vi "Autonomous Independent.vi"() -> ()   [LabVIEW 2016]
doc: "This VI is called when autonomous begins, and will automatically be terminated when autonomous ends. You can carry out timed or sensor driven robot movement independently without needing to return to the caller."
uses:
  <vilib>/Rock Robotics/Network Tables/NT Read Number.vi
  <vilib>/Rock Robotics/WPI/Solenoid/WPI_SolenoidValue.ctl
  Users/admin/Documents/Auto_Action_Typedef.ctl
panel:
  in  "Value":T1=enum."Forward"
  out "Auto Mode":dbl=3.0
  in  "Auton_Modes":T3(array[cluster])=[{"Actions"=[{"Effort"=0.55, "Duration"=3.5, "Action"=enum."Nothing"}, {"Effort"=0.0, "Duration"=0.0, "Action"=enum."Nothing"}]}, {"Actions"=[{"Effort"=0.0, "Duration"=1.0, "Action"=enum."Nothing"}, {"Effort"=0.75, "Duration"=5.0, "Action"=enum."Nothing"}, {"Effort"=0.0, "Duration"=1.0, "Action"=enum."Nothing"}]}, {"Actions"=[{"Effort"=1.0, "Duration"=3.0, "Action"=enum."Nothing"}, {"Effort"=0.0, "Duration"=1.0, "Action"=enum."Nothing"}, {"Effort"=0.75, "Duration"=3.5, "Action"=enum."Nothing"}, {"Effort"=0.0, "Duration"=1.0, "Action"=enum."Nothing"}]}, {"Actions"=[{"Effort"=0.0, "Duration"=0.5, "Action"=enum."Nothing"}, {"Effort"=0.8, "Duration"=5.28, "Action"=enum."Nothing"}, {"Effort"=0.0, "Duration"=1.0, "Action"=enum."Nothing"}, {"Effort"=-0.8, "Duration"=1.8, "Action"=enum."Nothing"}, {"Effort"=0.0, "Duration"=0.1, "Action"=enum."Nothing"}, {"Effort"=0.8, "Duration"=1.75, "Action"=enum."Nothing"}, {"Effort"=0.0, "Duration"=0.5, "Action"=enum."Nothing"}, {"Effort"=0.0, "Duration"=4.0, "Action"=enum."Nothing"}]}, {"Actions"=[{"Effort"=0.0, "Duration"=0.0, "Action"=enum."Nothing"}, {"Effort"=1.0, "Duration"=0.1, "Action"=enum."Nothing"}, {"Effort"=0.0, "Duration"=0.1, "Action"=enum."Nothing"}, {"Effort"=1.0, "Duration"=3.0, "Action"=enum."Nothing"}]}, {"Actions"=[{"Effort"=0.0, "Duration"=0.0, "Action"=enum."Nothing"}, {"Effort"=1.0, "Duration"=0.1, "Action"=enum."Nothing"}, {"Effort"=0.0, "Duration"=0.1, "Action"=enum."Nothing"}, {"Effort"=1.0, "Duration"=3.0, "Action"=enum."Nothing"}]}, {"Actions"=[{"Effort"=0.55, "Duration"=4.0, "Action"=enum."Nothing"}, {"Effort"=0.0, "Duration"=1.0, "Action"=enum."Nothing"}, {"Effort"=-0.5, "Duration"=0.6, "Action"=enum."Nothing"}, {"Effort"=0.75, "Duration"=1.0, "Action"=enum."Nothing"}, {"Effort"=0.0, "Duration"=1.0, "Action"=enum."Nothing"}, {"Effort"=0.75, "Duration"=3.0, "Action"=enum."Nothing"}]}, {"Actions"=[{"Effort"=0.0, "Duration"=0.5, "Action"=enum."Nothing"}, {"Effort"=0.55, "Duration"=4.25, "Action"=enum."Nothing"}, {"Effort"=0.0, "Duration"=0.0, "Action"=enum."Nothing"}, {"Effort"=0.0, "Duration"=0.3, "Action"=enum."Nothing"}, {"Effort"=0.9, "Duration"=2.0, "Action"=enum."Nothing"}]}, {"Actions"=[{"Effort"=0.0, "Duration"=0.0, "Action"=enum."Nothing"}]}]
  # "Nothing"
  # "Boiler Side Gear"
  # "Middle Gear"
  # "Farside Gear"
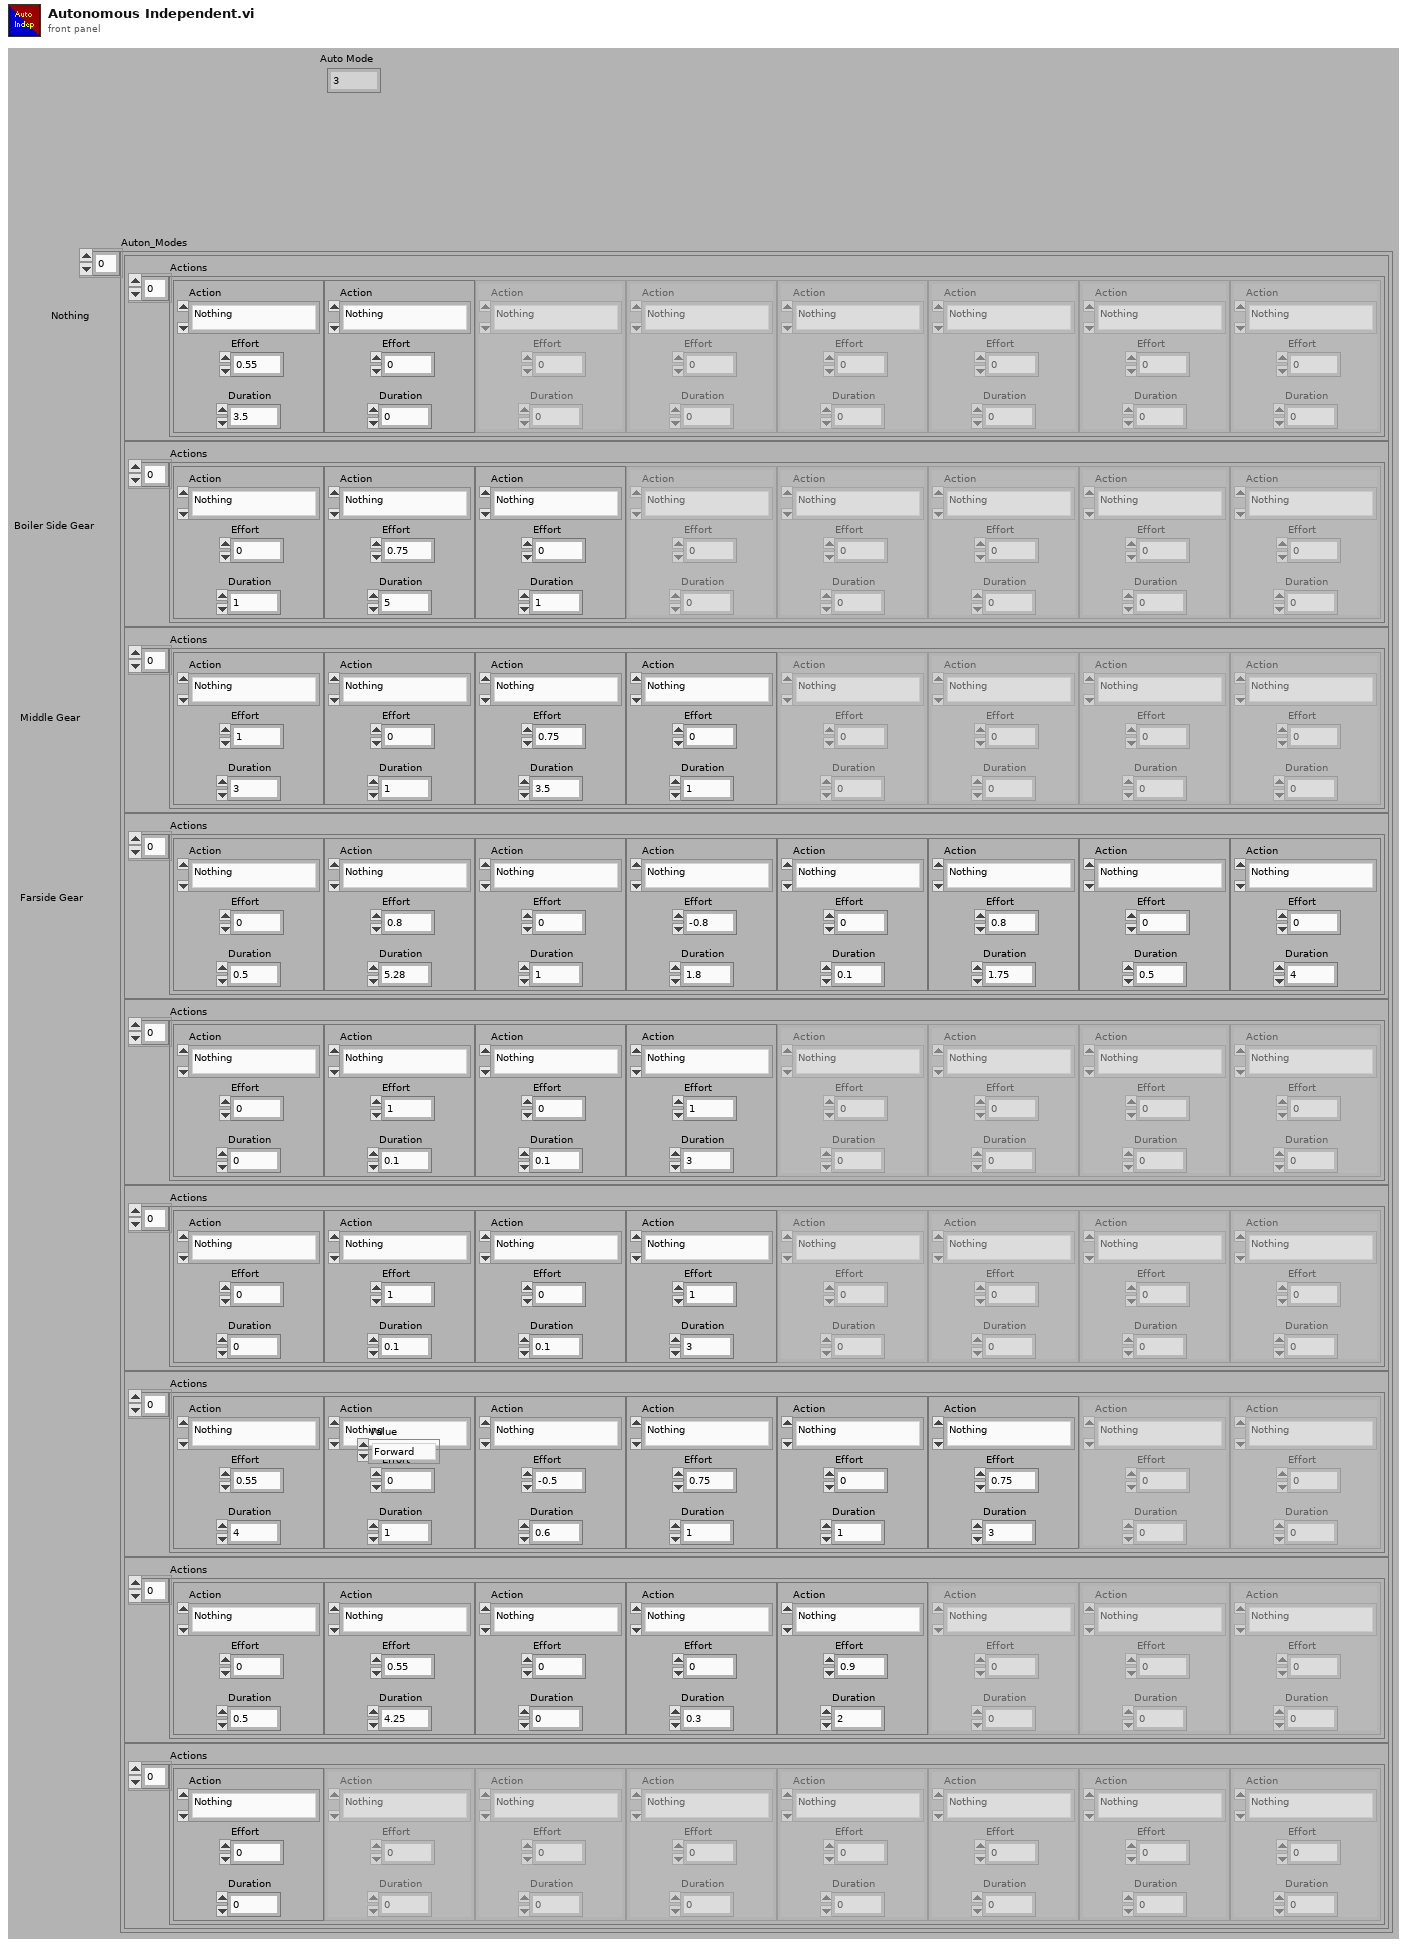
[diagram p1: front panel]
types:
  T1 = typedef "WPI_SolenoidValue.ctl" = enum16{"Off", "On", "Forward", "Reverse"}
  T2 = typedef "Auto_Action_Typedef.ctl" = enum16{"Nothing", "Drive", "Turn", "Gear0", "Gear1", "Climb", "Intake", "Index", "Shoot", "Test"}
  T3 = cluster{"Actions":cluster{"Effort":dbl, "Duration":dbl, "Action":T2}[]}[]
  T4 = cluster{"Actions":cluster{"Effort":dbl, "Duration":dbl, "Action":T2}[]}
  T5 = cluster{"Effort":dbl, "Duration":dbl, "Action":T2}[]
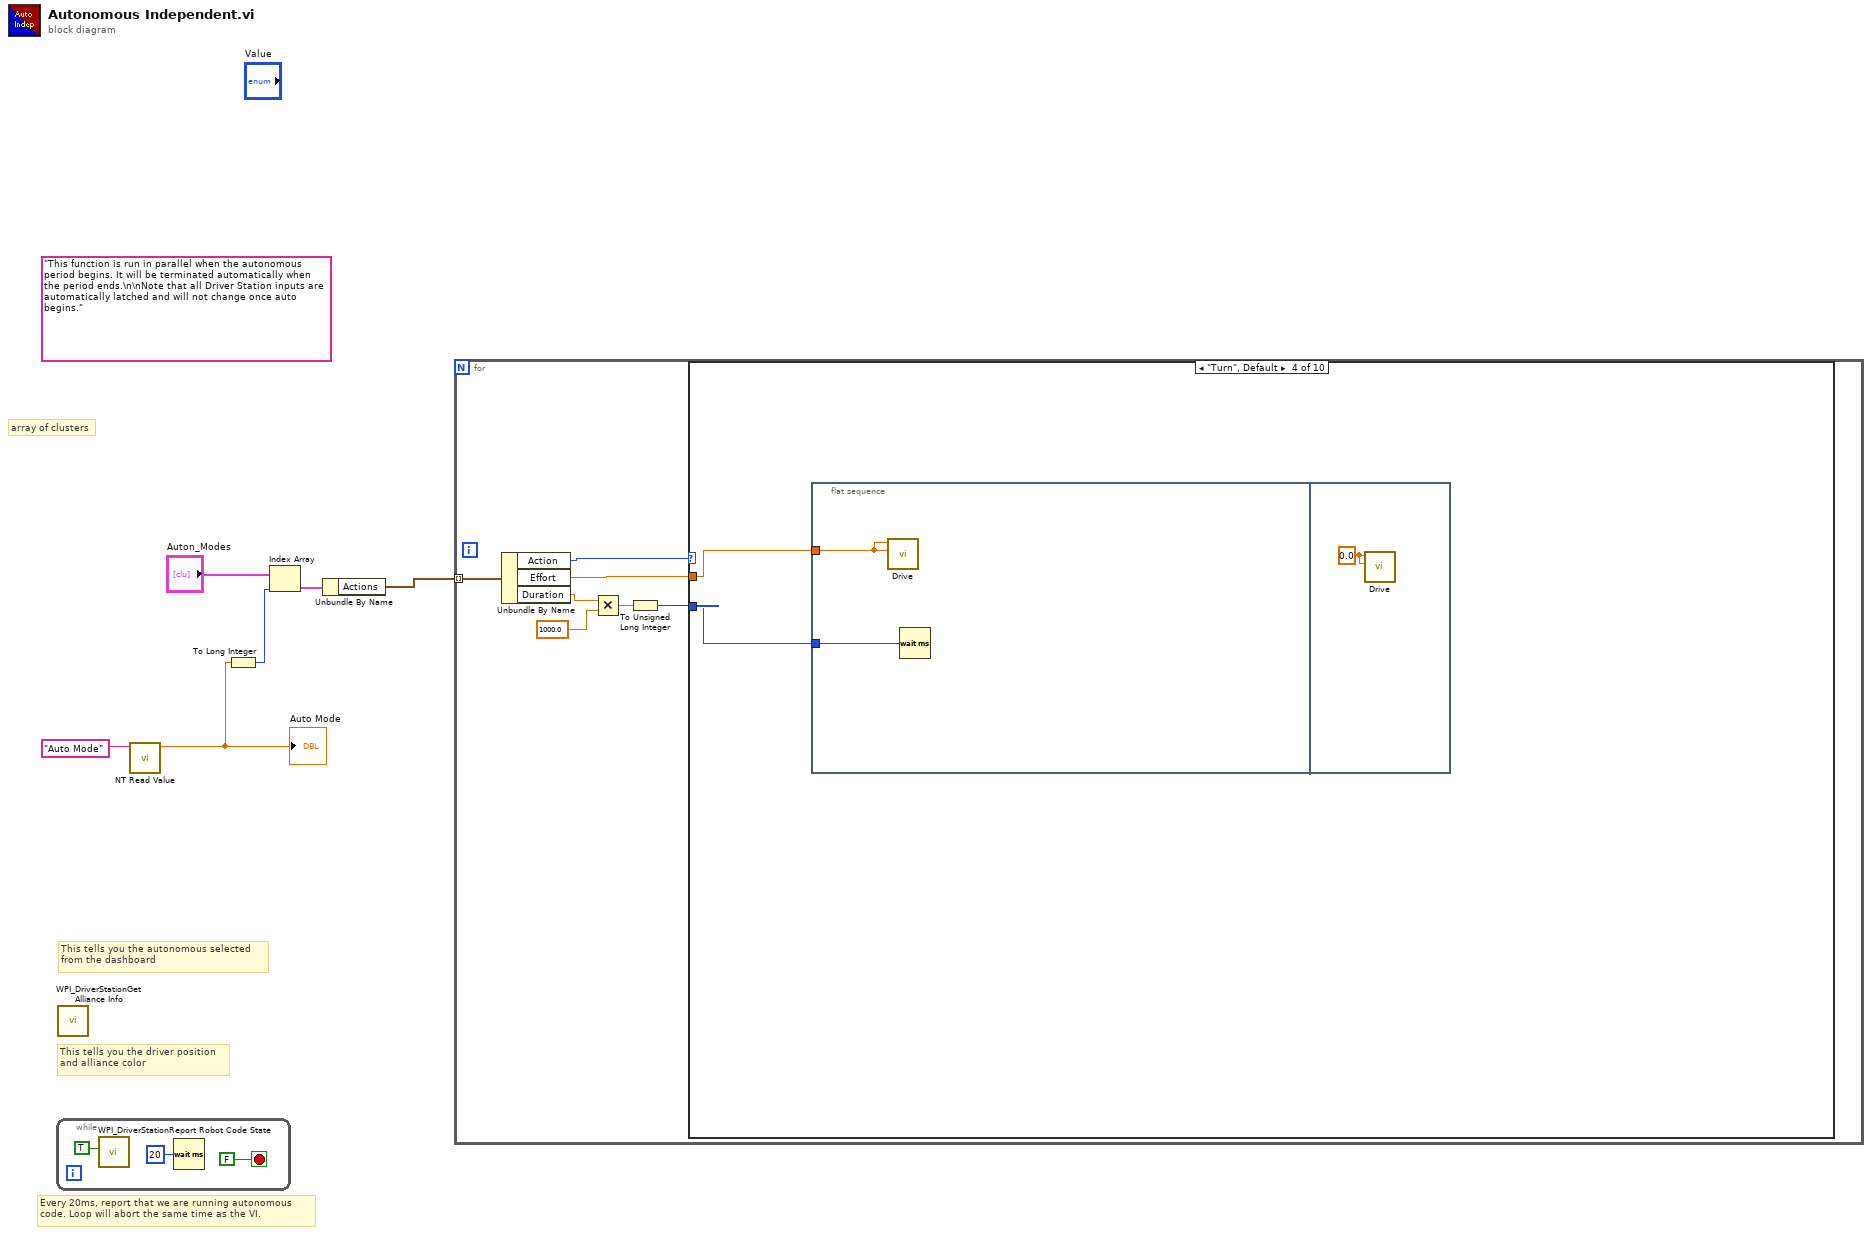
[diagram p0: block diagram]
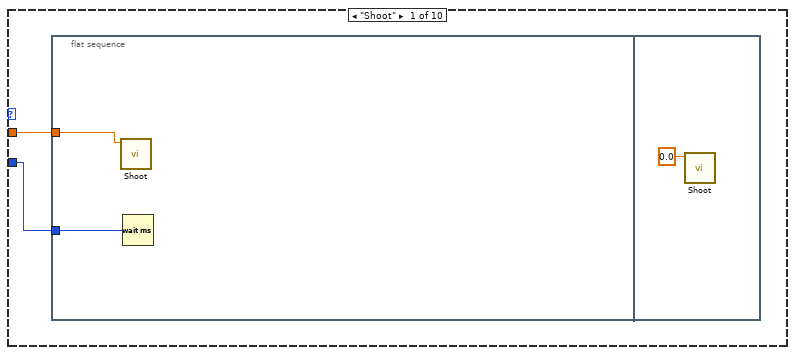
[diagram p2: hidden frame]
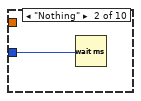
[diagram p3: hidden frame]
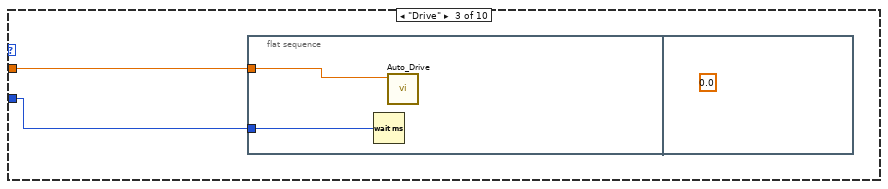
[diagram p4: hidden frame]
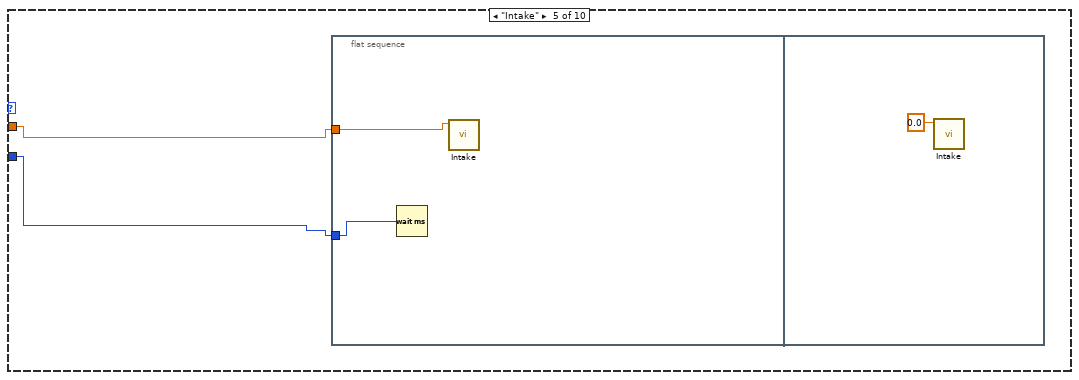
[diagram p5: hidden frame]
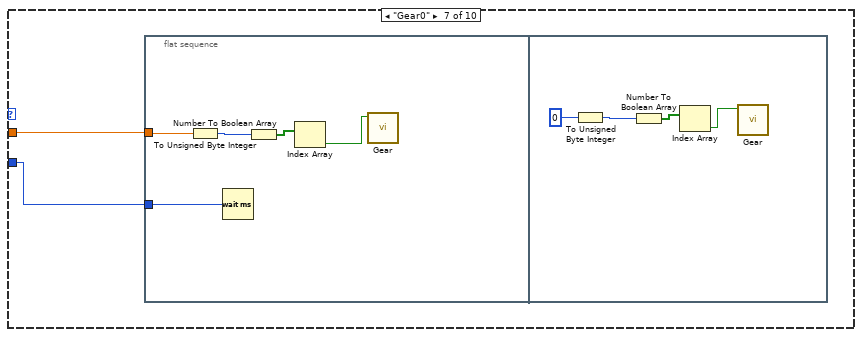
[diagram p7: hidden frame]
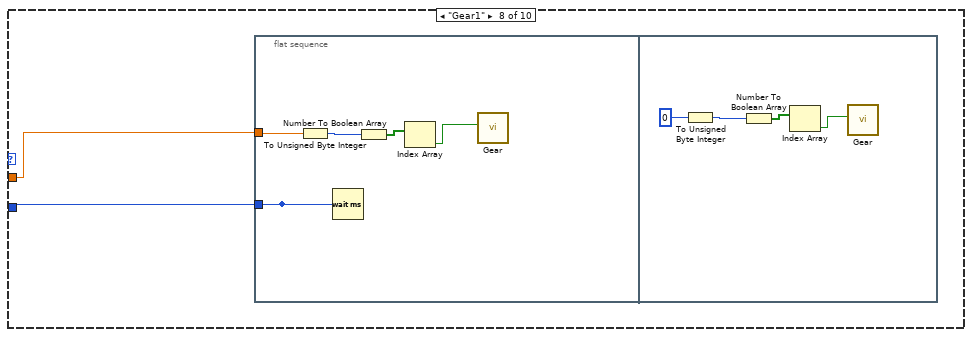
[diagram p8: hidden frame]
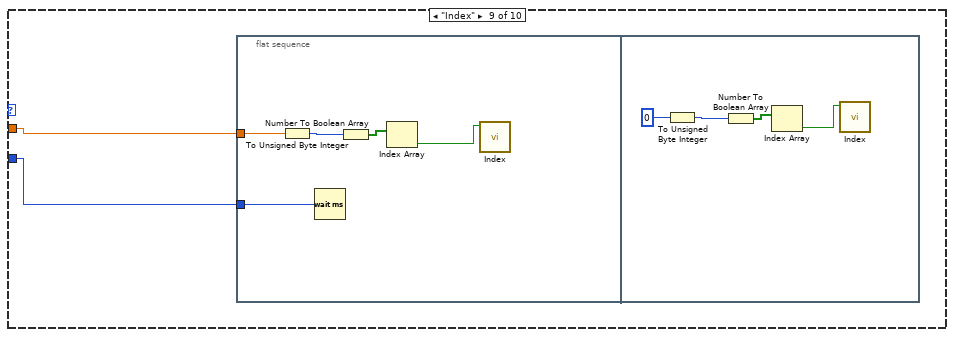
[diagram p9: hidden frame]
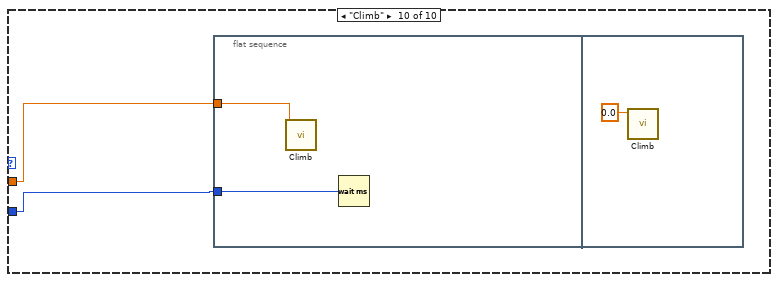
[diagram p10: hidden frame]
diagram:
  (unwired) "This function is run in parallel when the autonomous period begins. It will be terminated automatically when the period ends.\n\nNote that all Driver Station inputs are automatically latched and will not change once auto begins."
  # "This tells you the autonomous selected\nfrom the dashboard"
  # "array of clusters"
  # "Every 20ms, report that we are running autonomous\ncode. Loop will abort the same time as the VI."
  # "This tells you the driver position\nand alliance color"
  n1 = while {
    stop <- FALSE stop-if-true
    n2 = call <vilib>:"WPI_DriverStationReport Robot Code State.vi"("Autonomous"=TRUE) -> ()  [unwired: 10 in, 1 out]
    n3 = Wait (ms)(milliseconds to wait=u32 20) -> ()  [unwired: 1 out]
  }
  n4 = call <vilib>:"WPI_DriverStationGet Alliance Info.vi"() -> ()  [unwired: 12 out]
  n5 = call-poly <vilib>:"NT Read Value.vi"("Name"="Auto Mode") -> ("Numeric"=w1:dbl)  [unwired: 9 in, 1 out]
  "Auto Mode" <- w1
  n6 = To Long Integer(number=w1) -> (32bit integer=w3:i32)
  n7 = Index Array(array="Auton_Modes", index=w3) -> (element=w5:T4)
  n8 = Unbundle By Name(w5) -> ("Actions"=w6:T5)
  n9 = for {
    tunnel: w6 -> [w16] mode=indexing
    n10 = Unbundle By Name(w16) -> ("Action"=w15:T2, "Effort"=w14:dbl, "Duration"=w13:dbl)
    n11 = Multiply(x=w13, y=1000.0) -> (x*y=w11:dbl)
    n12 = To Unsigned Long Integer(number=w11) -> (unsigned 32bit integer=w10:u32)
    n13 = case shown="\"Turn\", Default" w15 {
      tunnel: w14 -> [w18 _ w24 w28 w33 _ w37 w49 w59 w71]
      tunnel: w10 -> [w17 w22 w23 w27 w32 _ w38 w48 w60 w70]
      frame "Shoot" {
        n14 = flat-sequence {
          tunnel: w18 -> [w20]
          tunnel: w17 -> [w19]
          frame #0 {
            n15 = call "Shoot.vi"("Effort"=w20) -> ()  [unwired: 11 in]
            n16 = Wait (ms)(milliseconds to wait=w19) -> ()  [unwired: 1 out]
          }
          frame #1 {
            n17 = call "Shoot.vi"("Effort"=0.0) -> ()  [unwired: 11 in]
          }
        }
      }
      frame "Nothing" {
        n18 = Wait (ms)(milliseconds to wait=w22) -> ()  [unwired: 1 out]
      }
      frame "Drive" {
        n19 = flat-sequence {
          tunnel: w24 -> [w25]
          tunnel: w23 -> [w26]
          frame #0 {
            n20 = Wait (ms)(milliseconds to wait=w26) -> ()  [unwired: 1 out]
            n21 = call "Auto_Drive.vi"(11:w25) -> ()  [unwired: 11 in]
          }
          frame #1 {
            (unwired) 0.0 ("Drive L")
          }
        }
      }
      frame "Turn", Default {
        n22 = flat-sequence {
          tunnel: w28 -> [w30]
          tunnel: w27 -> [w29]
          frame #0 {
            n23 = call "Drive.vi"("Drive R"=w30, "Drive L"=w30) -> ()  [unwired: 10 in]
            n24 = Wait (ms)(milliseconds to wait=w29) -> ()  [unwired: 1 out]
          }
          frame #1 {
            w31 = 0.0 ("Drive L")
            n25 = call "Drive.vi"("Drive R"=w31, "Drive L"=w31) -> ()  [unwired: 10 in]
          }
        }
      }
      frame "Intake" {
        n26 = flat-sequence {
          tunnel: w33 -> [w35]
          tunnel: w32 -> [w34]
          frame #0 {
            n27 = Wait (ms)(milliseconds to wait=w34) -> ()  [unwired: 1 out]
            n28 = call "Intake.vi"("Effort"=w35) -> ()  [unwired: 11 in]
          }
          frame #1 {
            n29 = call "Intake.vi"("Effort"=0.0) -> ()  [unwired: 11 in]
          }
        }
      }
      frame "Test" {
      }
      frame "Gear0" {
        n30 = flat-sequence {
          tunnel: w38 -> [w43]
          tunnel: w37 -> [w42]
          frame #0 {
            n31 = To Unsigned Byte Integer(number=w42) -> (unsigned 8bit integer=w41:u8)
            n32 = Wait (ms)(milliseconds to wait=w43) -> ()  [unwired: 1 out]
            n33 = Number To Boolean Array(number=w41) -> (Boolean array=w40:bool[])
            n34 = Index Array(array=w40) -> (element=w39:bool)  [unwired: 1 in]
            n35 = call "Gear.vi"("Gear0?"=w39) -> ()  [unwired: 11 in]
          }
          frame #1 {
            n36 = To Unsigned Byte Integer(number=u8 0) -> (unsigned 8bit integer=w46:u8)
            n37 = Number To Boolean Array(number=w46) -> (Boolean array=w47:bool[])
            n38 = Index Array(array=w47) -> (element=w44:bool)  [unwired: 1 in]
            n39 = call "Gear.vi"("Gear0?"=w44) -> ()  [unwired: 11 in]
          }
        }
      }
      frame "Gear1" {
        n40 = flat-sequence {
          tunnel: [w50] -> _
          tunnel: w49 -> [w54]
          tunnel: w48 -> [w50]
          frame #0 {
            n41 = To Unsigned Byte Integer(number=w54) -> (unsigned 8bit integer=w53:u8)
            n42 = Wait (ms)(milliseconds to wait=w50) -> ()  [unwired: 1 out]
            n43 = Number To Boolean Array(number=w53) -> (Boolean array=w52:bool[])
            n44 = Index Array(array=w52) -> (element=w51:bool)  [unwired: 1 in]
            n45 = call "Gear.vi"("Gear1?"=w51) -> ()  [unwired: 11 in]
          }
          frame #1 {
            n46 = To Unsigned Byte Integer(number=u8 0) -> (unsigned 8bit integer=w57:u8)
            n47 = Number To Boolean Array(number=w57) -> (Boolean array=w58:bool[])
            n48 = Index Array(array=w58) -> (element=w55:bool)  [unwired: 1 in]
            n49 = call "Gear.vi"("Gear1?"=w55) -> ()  [unwired: 11 in]
          }
        }
      }
      frame "Index" {
        n50 = flat-sequence {
          tunnel: w60 -> [w62]
          tunnel: w59 -> [w61]
          frame #0 {
            n51 = To Unsigned Byte Integer(number=w61) -> (unsigned 8bit integer=w65:u8)
            n52 = Wait (ms)(milliseconds to wait=w62) -> ()  [unwired: 1 out]
            n53 = Number To Boolean Array(number=w65) -> (Boolean array=w64:bool[])
            n54 = Index Array(array=w64) -> (element=w63:bool)  [unwired: 1 in]
            n55 = call "Index.vi"("Index?"=w63) -> ()  [unwired: 11 in]
          }
          frame #1 {
            n56 = To Unsigned Byte Integer(number=u8 0) -> (unsigned 8bit integer=w68:u8)
            n57 = Number To Boolean Array(number=w68) -> (Boolean array=w69:bool[])
            n58 = Index Array(array=w69) -> (element=w66:bool)  [unwired: 1 in]
            n59 = call "Index.vi"("Index?"=w66) -> ()  [unwired: 11 in]
          }
        }
      }
      frame "Climb" {
        n60 = flat-sequence {
          tunnel: w71 -> [w73]
          tunnel: w70 -> [w72]
          frame #0 {
            n61 = call "Climb.vi"("Effort"=w73) -> ()  [unwired: 11 in]
            n62 = Wait (ms)(milliseconds to wait=w72) -> ()  [unwired: 1 out]
          }
          frame #1 {
            n63 = call "Climb.vi"("Effort"=0.0) -> ()  [unwired: 11 in]
          }
        }
      }
    }
  }
